vi "Create G-CLI Script vipBuild.vi"(8 "error in (no error)":errorcluster, 10 "VIPB File Path":path, 11 "PostBuildSupport in":refnum<class "PostBuildSupport.lvclass">) -> (0 "error out":errorcluster, 2 "command":string, 3 "PostBuildSupport out":refnum<class "PostBuildSupport.lvclass">)   [LabVIEW 2019, in "PostBuildSupport.lvclass"]
uses:
  PostBuildSupport.lvclass
  PostBuildSupport.lvclass/PostBuildSupport.ctl
  VIPM/VIPM.lvlib
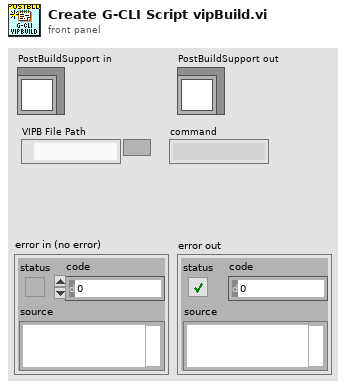
[diagram p1: front panel]
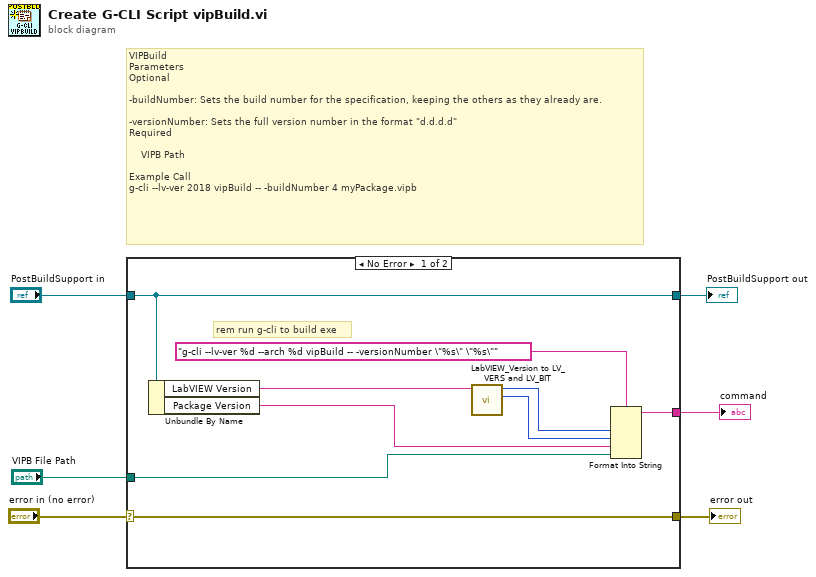
[diagram p0: block diagram]
diagram:
  # "VIPBuild\nParameters\nOptional\n\n-buildNumber: Sets the build number for the specification, keeping the others as they already are.\n\n-versionNumber: Sets the full version number in the format \"d.d.d.d\"\nRequired\n\n    VIPB Path\n\nExample Call\ng-cli --lv-ver 2018 vipBuild -- -buildNumber 4 myPackage.vipb"
  n1 = case shown="No Error" "error in (no error)" {
    selector: "error in (no error)" -> [w11 w17]
    tunnel: "PostBuildSupport in" -> [w15 w16]
    tunnel: [w11 w17] -> w4
    tunnel: [w15 w16] -> w3
    tunnel: [w12 _] -> w2
    tunnel: "VIPB File Path" -> [w10 _]
    frame No Error {
      # "rem run g-cli to build exe"
      n2 = Unbundle By Name(w15) -> ("LabVIEW Version"=w9:string, "Package Version"=w13:string)
      n3 = call "LabVIEW_Version to LV_VERS and LV_BIT.vi"("Package_LabVIEW_Version"=w9) -> ("LV_BIT"=w7:u32, "LV_VER"=w8:u32)  [unwired: 9 in]
      n4 = Format Into String(format string="g-cli --lv-ver %d --arch %d vipBuild -- -versionNumber \"%s\" \"%s\"", w8, w7, w13, w10) -> (resulting string=w12:string)  [unwired: 2 in, 1 out]
    }
    frame Error {
    }
  }
  "error out" <- w4
  "PostBuildSupport out" <- w3
  "command" <- w2
